vi "testmethod.vi"   [LabVIEW 2009]
uses:
  Planet/Planet.lvclass
  Enumerations/PlanetNameValues.ctl
  Difftrack/DifftrackRADec/DifftrackRADec.lvclass
  Target.lvclass
types:
  T1 = typedef "PlanetNameValues.ctl" = enum16{"Mercury", "Venus", "Moon", "Mars", "Jupiter", "Saturn", "Uranus", "Neptune", "Pluto"}
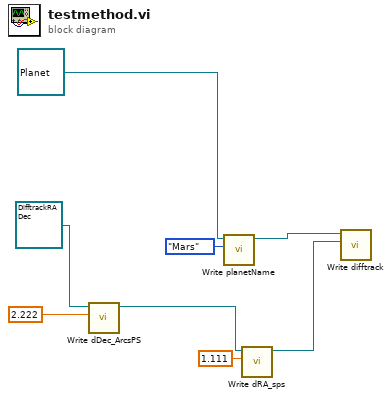
[diagram p0: block diagram]
diagram:
  n1 = call "Write dDec_ArcsPS.vi"("dDec_ArcsPS"=dbl[unit] 2.222, "DifftrackRADec in"=refnum<class "DifftrackRADec.lvclass"> refnum ("DifftrackRADec.lvclass")) -> ("DifftrackRADec out"=w2:refnum<class "DifftrackRADec.lvclass">)  [unwired: 8 in, 1 out]
  n2 = call "Write planetName.vi"("planetName"=PlanetNameValues."Mars", "Planet in"=refnum<class "Planet.lvclass"> refnum) -> ("Planet out"=w6:refnum<class "Planet.lvclass">)  [unwired: 8 in, 1 out]
  n3 = call "Write dRA_sps.vi"("dRA_sps"=1.111, "DifftrackRADec in"=w2) -> ("DifftrackRADec out"=w1:refnum<class "DifftrackRADec.lvclass">)  [unwired: 8 in, 1 out]
  n4 = call "Write difftrack.vi"("Difftrack.lvclass"=w1, "Target in"=w6) -> ()  [unwired: 8 in, 2 out]
